vi "SQL Insert Table.vi"(8 "error in (no error)":errorcluster, 10 "SQLite Connection in":refnum<class "Connection.lvclass">, 11 "variant":variant) -> (0 "error out":errorcluster, 3 "SQLite Connection":refnum<class "Connection.lvclass">)   [LabVIEW 2021]
uses:
  <vilib>/Utility/Data Type/Type Definitions/Data Type.ctl
  <vilib>/drjdpowell/SQLite Library/SQL Connection/Connection.lvclass
  <vilib>/drjdpowell/SQLite Library/SQL Connection/Execute SQL (Variant Cluster results).vi
  <vilib>/Utility/Data Type/NI_Data Type.lvlib
  <vilib>/drjdpowell/SQLite Library/SQLite.lvlib
panel:
  out "Insert Statement":string
  out "Array":T2(array[cluster])
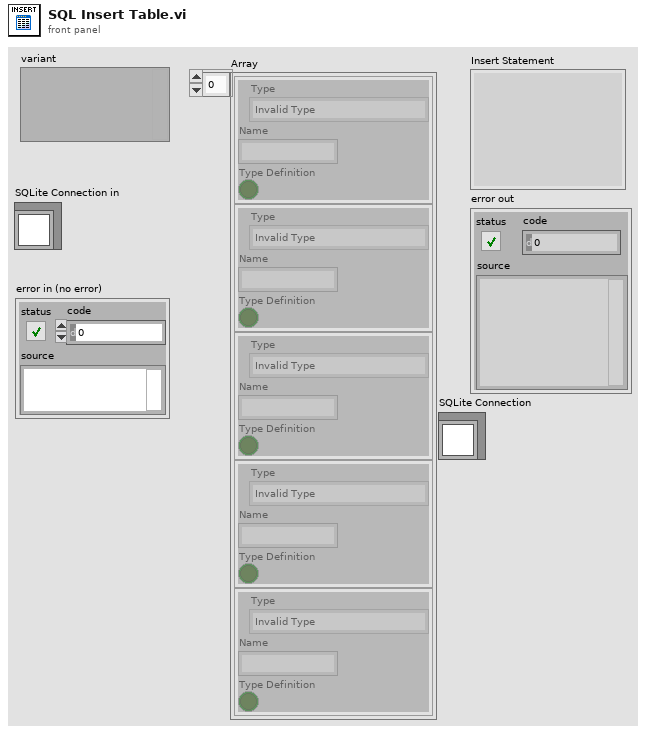
[diagram p1: front panel]
types:
  T1 = typedef "NI_Data Type.lvlib/Data Type.ctl" = enum8{"Invalid Type", "Void", "I8", "I16", "I32", "I64", "U8", "U16", "U32", "U64", "Single Float", "Double Float", "Extended Float", "Single Complex", "Double Complex", "Extended Complex", "Enum U8", "Enum U16", "Enum U32", "Enum U64", "Single Float With Unit", "Double Float With Unit", "Extended Float With Unit", "Single Complex with Unit", "Double Complex with Unit", "Extended Complex with Unit", "Boolean", "String", "Path", "Picture", "Tag", "Array", "Cluster", "Variant", "LV Variant", "Waveform", "Timestamp", "Digital Waveform", "Digital Data", "ExpressData", "Refnum", "External Data", "VI", "Poly VI", "LabVIEW Class Instance", "Fixed Point", "Set Collection", "Map Collection"}
  T2 = cluster{"Type":T1, "Name":string, "Type Definition":bool}[]
  T3 = cluster{"type":T1, "name":string, "type definition":bool}
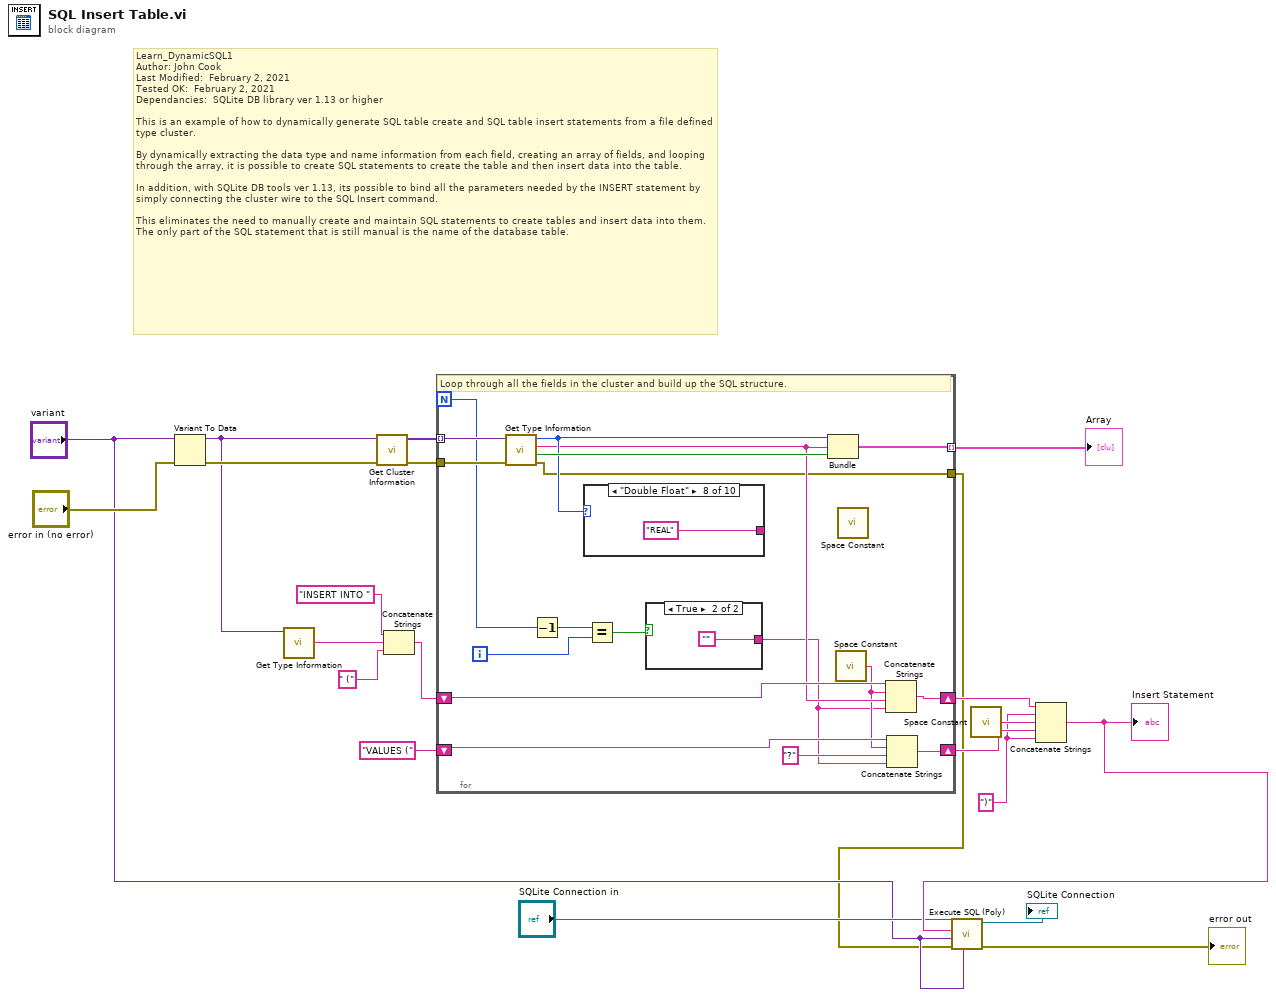
[diagram p0: block diagram]
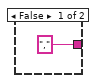
[diagram p2: hidden frame]
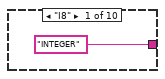
[diagram p3: hidden frame]
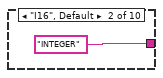
[diagram p4: hidden frame]
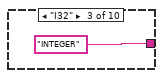
[diagram p5: hidden frame]
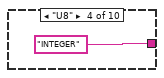
[diagram p6: hidden frame]
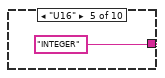
[diagram p7: hidden frame]
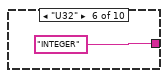
[diagram p8: hidden frame]
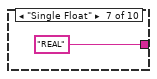
[diagram p9: hidden frame]
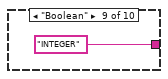
[diagram p10: hidden frame]
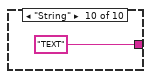
[diagram p11: hidden frame]
diagram:
  w12 = ")"
  # "Learn_DynamicSQL1\nAuthor: John Cook\nLast Modified:  February 2, 2021\nTested OK:  February 2, 2021\nDependancies:  SQLite DB library ver 1.13 or higher\n\nThis is an example of how to dynamically generate SQL table create and SQL table insert statements from a file defined type cluster.\n\nBy dynamically extracting the data type and name information from each field, creating an array of fields, and looping through the array, it is possible to create SQL statements to create the table and then insert data into the table.\n\nIn addition, with SQLite DB tools ver 1.13, its possible to bind all the parameters needed by the INSERT statement by simply connecting the cluster wire to the SQL Insert command.\n\nThis eliminates the need to manually create and maintain SQL statements to create tables and insert data into them.  The only part of the SQL statement that is still manual is the name of the database table."
  n1 = Variant To Data(error in="error in (no error)", Variant="variant") -> (data=w7:variant, error out=w21:errorcluster)  [unwired: 1 in]
  n2 = call <vilib>:"Get Type Information.vi"("variant"=w7) -> ("name"=w5:string)  [unwired: 6 in, 4 out]
  n3 = call <vilib>:"Get Cluster Information.vi"("error in (no error)"=w21, "variant"=w7) -> ("error out"=w19:errorcluster, "cluster elements"=w20:variant[])  [unwired: 8 in]
  n4 = Concatenate Strings("INSERT INTO ", w5, " (") -> (w3:string)
  n5 = for {
    N -> [w32]
    tunnel: w20 -> [w36] mode=indexing
    tunnel: w19 -> [w39]
    tunnel: [w37] -> w17 mode=indexing
    shift-right: [w30] -> w13
    shift-left: w3 -> [w29]
    shift-right: [w26] -> w14
    shift-left: "VALUES (" -> [w27]
    tunnel: [w23] -> w8
    i -> [w34]
    # "Loop through all the fields in the cluster and build up the SQL structure."
    n6 = call <vilib>:"Get Type Information.vi"("error in (no error)"=w39, "variant"=w36) -> ("error out"=w23:errorcluster, "type definition"=w38:bool, "name"=w28:string, "type"=w35:T1)  [unwired: 5 in, 1 out]
    n7 = Decrement(x=w32) -> (x-1=w31:i32)
    n8 = case shown="\"Double Float\"" w35 {
      tunnel: ["INTEGER" "INTEGER" "INTEGER" "INTEGER" "INTEGER" "INTEGER" "REAL" "REAL" "INTEGER" "TEXT"] -> _
      frame "I8" {
      }
      frame "I16", Default {
      }
      frame "I32" {
      }
      frame "U8" {
      }
      frame "U16" {
      }
      frame "U32" {
      }
      frame "Single Float" {
      }
      frame "Double Float" {
      }
      frame "Boolean" {
      }
      frame "String" {
      }
    }
    n9 = Equal?(x=w31, y=w34) -> (x = y?=w33:bool)
    n10 = case shown="True" w33 {
      tunnel: ["," ("delimiter (Tab)") ""] -> w22
      frame False {
      }
      frame True {
      }
    }
    n11 = Bundle("type"=w35, "name"=w28, "type definition"=w38) -> (w37:T3)  [unwired: 1 in]
    n12 = call <vilib>:"Space Constant.vi"() -> ("String"=w25:string)
    n13 = call <vilib>:"Space Constant.vi"() -> ()  [unwired: 1 out]
    n14 = Concatenate Strings(w29, w25, w28, w22) -> (w30:string)
    n15 = Concatenate Strings(w27, w25, "?" ("string"), w22) -> (w26:string)
  }
  "Array" <- w17
  n16 = call <vilib>:"Space Constant.vi"() -> ("String"=w15:string)
  n17 = Concatenate Strings(w13, w12, w15, w14, w12) -> (w11:string)
  "Insert Statement" <- w11
  n18 = call-poly <vilib>:"Execute SQL (Poly).vi"("Parameter(s)"="variant", "error in (no error)"=w8, "Cluster"="variant", "SQL"=w11, "SQLite Connection in"="SQLite Connection in") -> ("error out"=→"error out":errorcluster, "SQLite Connection"=→"SQLite Connection":refnum<class "Connection.lvclass">)  [unwired: 4 in, 1 out]
